vi "Configure CVD Alpha Conversion.vi"(0 "VISA resource name":refnum<visa-resource-name>, 1 "Rzero value (100)":dbl=100.0, 5 "Probe Identity (Probe1)":string="Probe1", 7 "Connection (0: Two wire)":u16(ring) items=["Two wire", "Three wire", "Four wire"], 11 "error in (no error)":errorcluster, 12 "alpha value (0.00385055)":dbl=0.00385055 format="%#_10g", 13 "beta value (-0.10863432)":dbl=-0.10863432 format="%#_10g", 14 "delta value (1.499785745)":dbl=1.499785745 format="%#_10g") -> (4 "VISA resource name out":refnum<visa-resource-name>, 15 "error out":errorcluster)   [LabVIEW 2011, in "Fluke 8508.lvlib"]
doc: "This VI configures a new probe or sets an existing one for CVD alpha conversion for a temperature reading.\n\nNOTE:\nThis VI merely configures the probe and will not set the PRT function on the instrument. In order to set the function, run the Configure Temperature VI after running this VI."
uses:
  Fluke 8508.lvlib
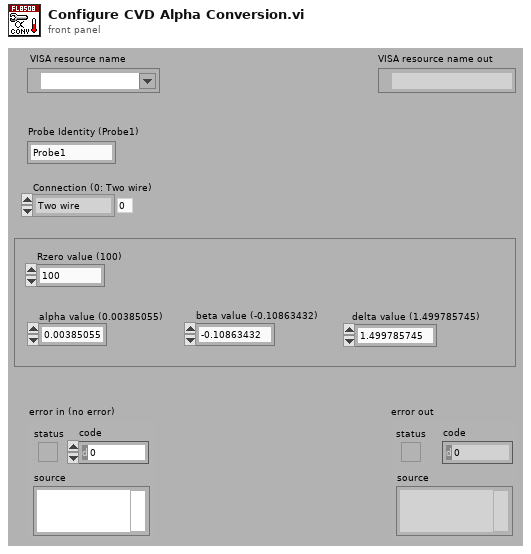
[diagram p1: front panel]
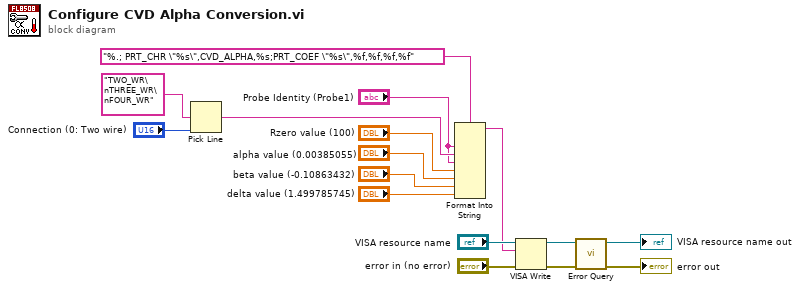
[diagram p0: block diagram]
diagram:
  n1 = Pick Line(multi-line string="TWO_WR\nTHREE_WR\nFOUR_WR", line index="Connection (0: Two wire)") -> (output string=w8:string)  [unwired: 1 in]
  n2 = Format Into String(format string="%.; PRT_CHR \"%s\",CVD_ALPHA,%s;PRT_COEF \"%s\",%f,%f,%f,%f", "Probe Identity (Probe1)", w8, "Probe Identity (Probe1)", "Rzero value (100)", "alpha value (0.00385055)", "beta value (-0.10863432)", "delta value (1.499785745)") -> (resulting string=w10:string)  [unwired: 2 in, 1 out]
  n3 = VISA Write(VISA resource name="VISA resource name", write buffer=w10, error in (no error)="error in (no error)") -> (VISA resource name out=w2:refnum<visa-resource-name>, error out=w4:errorcluster)  [unwired: 1 out]
  n4 = call "Error Query.vi"("error in (no error)"=w4, "VISA resource name"=w2) -> ("error out"=→"error out":errorcluster, "VISA resource name out"=→"VISA resource name out":refnum<visa-resource-name>)  [unwired: 6 in, 2 out]
